vi "Defaults.vi"() -> (3 "TVC Data":T6={"UI References"={"Exit Ref"=refnum, "Save Ref"=refnum, "Export Ref"=refnum, "Acquire Ref"=refnum, "Configure Ref"=refnum, "Graph Ref"=refnum, "Analyze Ref"=refnum, "Status Ref"=refnum, "Snapshot Ref"=refnum, "Start Ref"=refnum}, "User Specified"={"Hardware Configuration"={"VGC50"={"serial settings"={"port"="Inficon_VGC503", "baud rate"=115200}, "device information"={"type"="", "model number"="", "serial number"="", "firmware version"="", "hardware version"=""}, "VGC"=refnum, "Backing SP"={"mode"=2, "thresholds"={"lower"=0.0001, "upper"=0.005}, "on"=FALSE}, "Chamber SP"={"mode"=3, "thresholds"={"lower"=1e-05, "upper"=0.0001}, "on"=FALSE}}, "PTC10"={"serial settings"={"port"="Stanford_PTC10", "baud rate"=9600}, "PTC10 Info"={"Manufacturer"="", "Instrument"="", "Serial Number"="", "Firmware"=""}, "VISA resource name"="", "pwmloop"="define pwmloop(#t=0 while (1) {waitforsample if(#pwm=0){relays=0}else{if(#t<#pwm) {relays=1}else{relays=3}}#t+=1 if  (#t>99){#t=0} pause 0.2 s})", "onecycle"="define onecycle (pwm=100 run pwmloop 5A.PID.Setpoint=-130.0 5A.PID.input=3C while(#3C>-129.0){pause 0.2 s}pwm=-130 pause 10 min pwm=0  5A.PID.SetPoint=50.0 while(#3C<49.0){pause 0.2 s} pause 10 min kill pwmloop)", "control"="define control (while (#Cycles>0) {onecycle pause 1 s #Cycles-=1})", "HeatDrive"="define Failsafe (while(1) {if (#Check <-20){relays=0 outputEnable Off}else{if(#Check>20){relays=0 outputEnable Off}} pause 1 s})", "ToAmbient"="define ToAmbient(if(#3C>25.0){pwm=100 run pwmloop while(#3C>#25.0){pause 0.5 s} pwm=0 kill pwmloop}else{#5A.PID.setpoint=20.0 while(#3C<15.0){pause 0.5 s} outputenable off})", "StartupCode"="system.display.Monitors Show", "LogChannels"=[], "Heater O/P Channel"="", " Control Input"="", "TAmbient"=1.14, "AmbientTolerance"=0.012, "TestCycleParameters"={"TAmb"=20.0, "HeaterTestTemp"=51.5, "HeaterTestDwell(min)"=20, "HeaterTestDuration"=20, "MinOpTemp"=1.0, "MinOpDwell(min)"=1, "TestHeatingRate (deg/min)"=-131.5, "SurviveCycleParameters"={"MinSurviveTemp"=-131.5, "MinSurvive Dwell(min)"=10, "MaxSurviveTemp"=50.0, "MaxSurviveDwell(min)"=30, "ControlInput"=2, "ColdStandOff"=4.0, "HotStandoff"=5.0, "SteadyPWM"=20, "MaxCoolingRate (deg/min)"=3.75, "MaxHeatingRate (deg/min)"=2.5}, "CycleType"=0, "MaxOpTemp"=-50.0, "MinOpDwell(min)"=30}, "PID Params"={"P"=1.14, "I"=0.012, "D"=21.68, "Set"=0.0}}}, "Vacuum Graph config"={"Log/Lin"=FALSE, "Show Backing"=FALSE, "Show Chamber"=FALSE}}} {"User Specified"."Hardware Configuration"."PTC10"."PID Params"."D" min=0.0; "User Specified"."Hardware Configuration"."PTC10"."PID Params"."I" min=0.0; "User Specified"."Hardware Configuration"."PTC10"."PID Params"."P" min=0.0; "User Specified"."Hardware Configuration"."PTC10"."TestCycleParameters"."CycleType" items=["Survival", "Operational"]; "User Specified"."Hardware Configuration"."PTC10"."TestCycleParameters"."SurviveCycleParameters"."SteadyPWM" min=0 max=100 step=1; "User Specified"."Hardware Configuration"."PTC10"."serial settings"."baud rate" items=["9600"=9600, "19200"=19200, "38400"=38400, "57600"=57600, "115200"=115200]; "User Specified"."Hardware Configuration"."VGC50"."Chamber SP"."thresholds"."upper" format="%#_5p"; "User Specified"."Hardware Configuration"."VGC50"."Chamber SP"."thresholds"."lower" format="%#_5p"; "User Specified"."Hardware Configuration"."VGC50"."Chamber SP"."mode" items=["off", "on", "channel 1", "channel 2", "channel 3"]; "User Specified"."Hardware Configuration"."VGC50"."Backing SP"."thresholds"."upper" format="%#_5p"; "User Specified"."Hardware Configuration"."VGC50"."Backing SP"."thresholds"."lower" format="%#_5p"; "User Specified"."Hardware Configuration"."VGC50"."Backing SP"."mode" items=["off", "on", "channel 1", "channel 2", "channel 3"]; "User Specified"."Hardware Configuration"."VGC50"."serial settings"."baud rate" items=["9600"=9600, "19200"=19200, "38400"=38400, "57600"=57600, "115200"=115200]})   [LabVIEW 2024]
uses:
  controls/VGC50.ctl
  <instrlib>/PL Inficon VGC/PL Inficon VGC.lvclass
  controls/Data.ctl
  controls/UI References.ctl
  controls/User Specified Data.ctl
  controls/HW Configuration.ctl
  controls/SRS PTC10.ctl
  controls/TestCycleParams.ctl
  controls/SurviveCycleParams.ctl
  controls/ControlInput.ctl
  controls/PID Params.ctl
  controls/Vac Graph Config.ctl
panel:
  in  "PTC10":T1={"serial settings"={"port"="Stanford_PTC10", "baud rate"=9600}, "PTC10 Info"={"Manufacturer"="", "Instrument"="", "Serial Number"="", "Firmware"=""}, "VISA resource name"="", "pwmloop"="define pwmloop(#t=0 while (1) {waitforsample if(#pwm=0){relays=0}else{if(#t<#pwm) {relays=1}else{relays=3}}#t+=1 if  (#t>99){#t=0} pause 0.2 s})", "onecycle"="define onecycle (pwm=100 run pwmloop 5A.PID.Setpoint=-130.0 5A.PID.input=3C while(#3C>-129.0){pause 0.2 s}pwm=-130 pause 10 min pwm=0  5A.PID.SetPoint=50.0 while(#3C<49.0){pause 0.2 s} pause 10 min kill pwmloop)", "control"="define control (while (#Cycles>0) {onecycle pause 1 s #Cycles-=1})", "HeatDrive"="define Failsafe (while(1) {if (#Check <-20){relays=0 outputEnable Off}else{if(#Check>20){relays=0 outputEnable Off}} pause 1 s})", "ToAmbient"="define ToAmbient(if(#3C>25.0){pwm=100 run pwmloop while(#3C>#25.0){pause 0.5 s} pwm=0 kill pwmloop}else{#5A.PID.setpoint=20.0 while(#3C<15.0){pause 0.5 s} outputenable off})", "StartupCode"="system.display.Monitors Show", "LogChannels"=[], "Heater O/P Channel"="", " Control Input"="", "TAmbient"=20.0, "AmbientTolerance"=5.0, "TestCycleParameters"={"TAmb"=20.0, "HeaterTestTemp"=-80.0, "HeaterTestDwell(min)"=30, "HeaterTestDuration"=15, "MinOpTemp"=-50.0, "MinOpDwell(min)"=30, "TestHeatingRate (deg/min)"=0.4, "SurviveCycleParameters"={"MinSurviveTemp"=-131.5, "MinSurvive Dwell(min)"=10, "MaxSurviveTemp"=50.0, "MaxSurviveDwell(min)"=30, "ControlInput"=2, "ColdStandOff"=4.0, "HotStandoff"=5.0, "SteadyPWM"=20, "MaxCoolingRate (deg/min)"=3.75, "MaxHeatingRate (deg/min)"=2.5}, "CycleType"=0, "MaxOpTemp"=-50.0, "MinOpDwell(min)"=30}, "PID Params"={"P"=1.14, "I"=0.012, "D"=21.68, "Set"=0.0}} {"PID Params"."D" min=0.0; "PID Params"."I" min=0.0; "PID Params"."P" min=0.0; "TestCycleParameters"."CycleType" items=["Survival", "Operational"]; "TestCycleParameters"."SurviveCycleParameters"."SteadyPWM" min=0 max=100 step=1; "TestCycleParameters"."SurviveCycleParameters"."ControlInput" items=["3A", "3B", "3C", "3D", "4A", "4B", "4C", "4D"]; "serial settings"."baud rate" items=["9600"=9600, "19200"=19200, "38400"=38400, "57600"=57600, "115200"=115200]}
  in  "VGC50":T10={"serial settings"={"port"="Inficon_VGC503", "baud rate"=115200}, "device information"={"type"="", "model number"="", "serial number"="", "firmware version"="", "hardware version"=""}, "VGC"=refnum, "Backing SP"={"mode"=2, "thresholds"={"lower"=0.0001, "upper"=0.005}, "on"=FALSE}, "Chamber SP"={"mode"=3, "thresholds"={"lower"=1e-05, "upper"=0.0001}, "on"=FALSE}} {"Chamber SP"."thresholds"."upper" format="%#_5p"; "Chamber SP"."thresholds"."lower" format="%#_5p"; "Chamber SP"."mode" items=["off", "on", "channel 1", "channel 2", "channel 3"]; "Backing SP"."thresholds"."upper" format="%#_5p"; "Backing SP"."thresholds"."lower" format="%#_5p"; "Backing SP"."mode" items=["off", "on", "channel 1", "channel 2", "channel 3"]; "serial settings"."baud rate" items=["9600"=9600, "19200"=19200, "38400"=38400, "57600"=57600, "115200"=115200]}
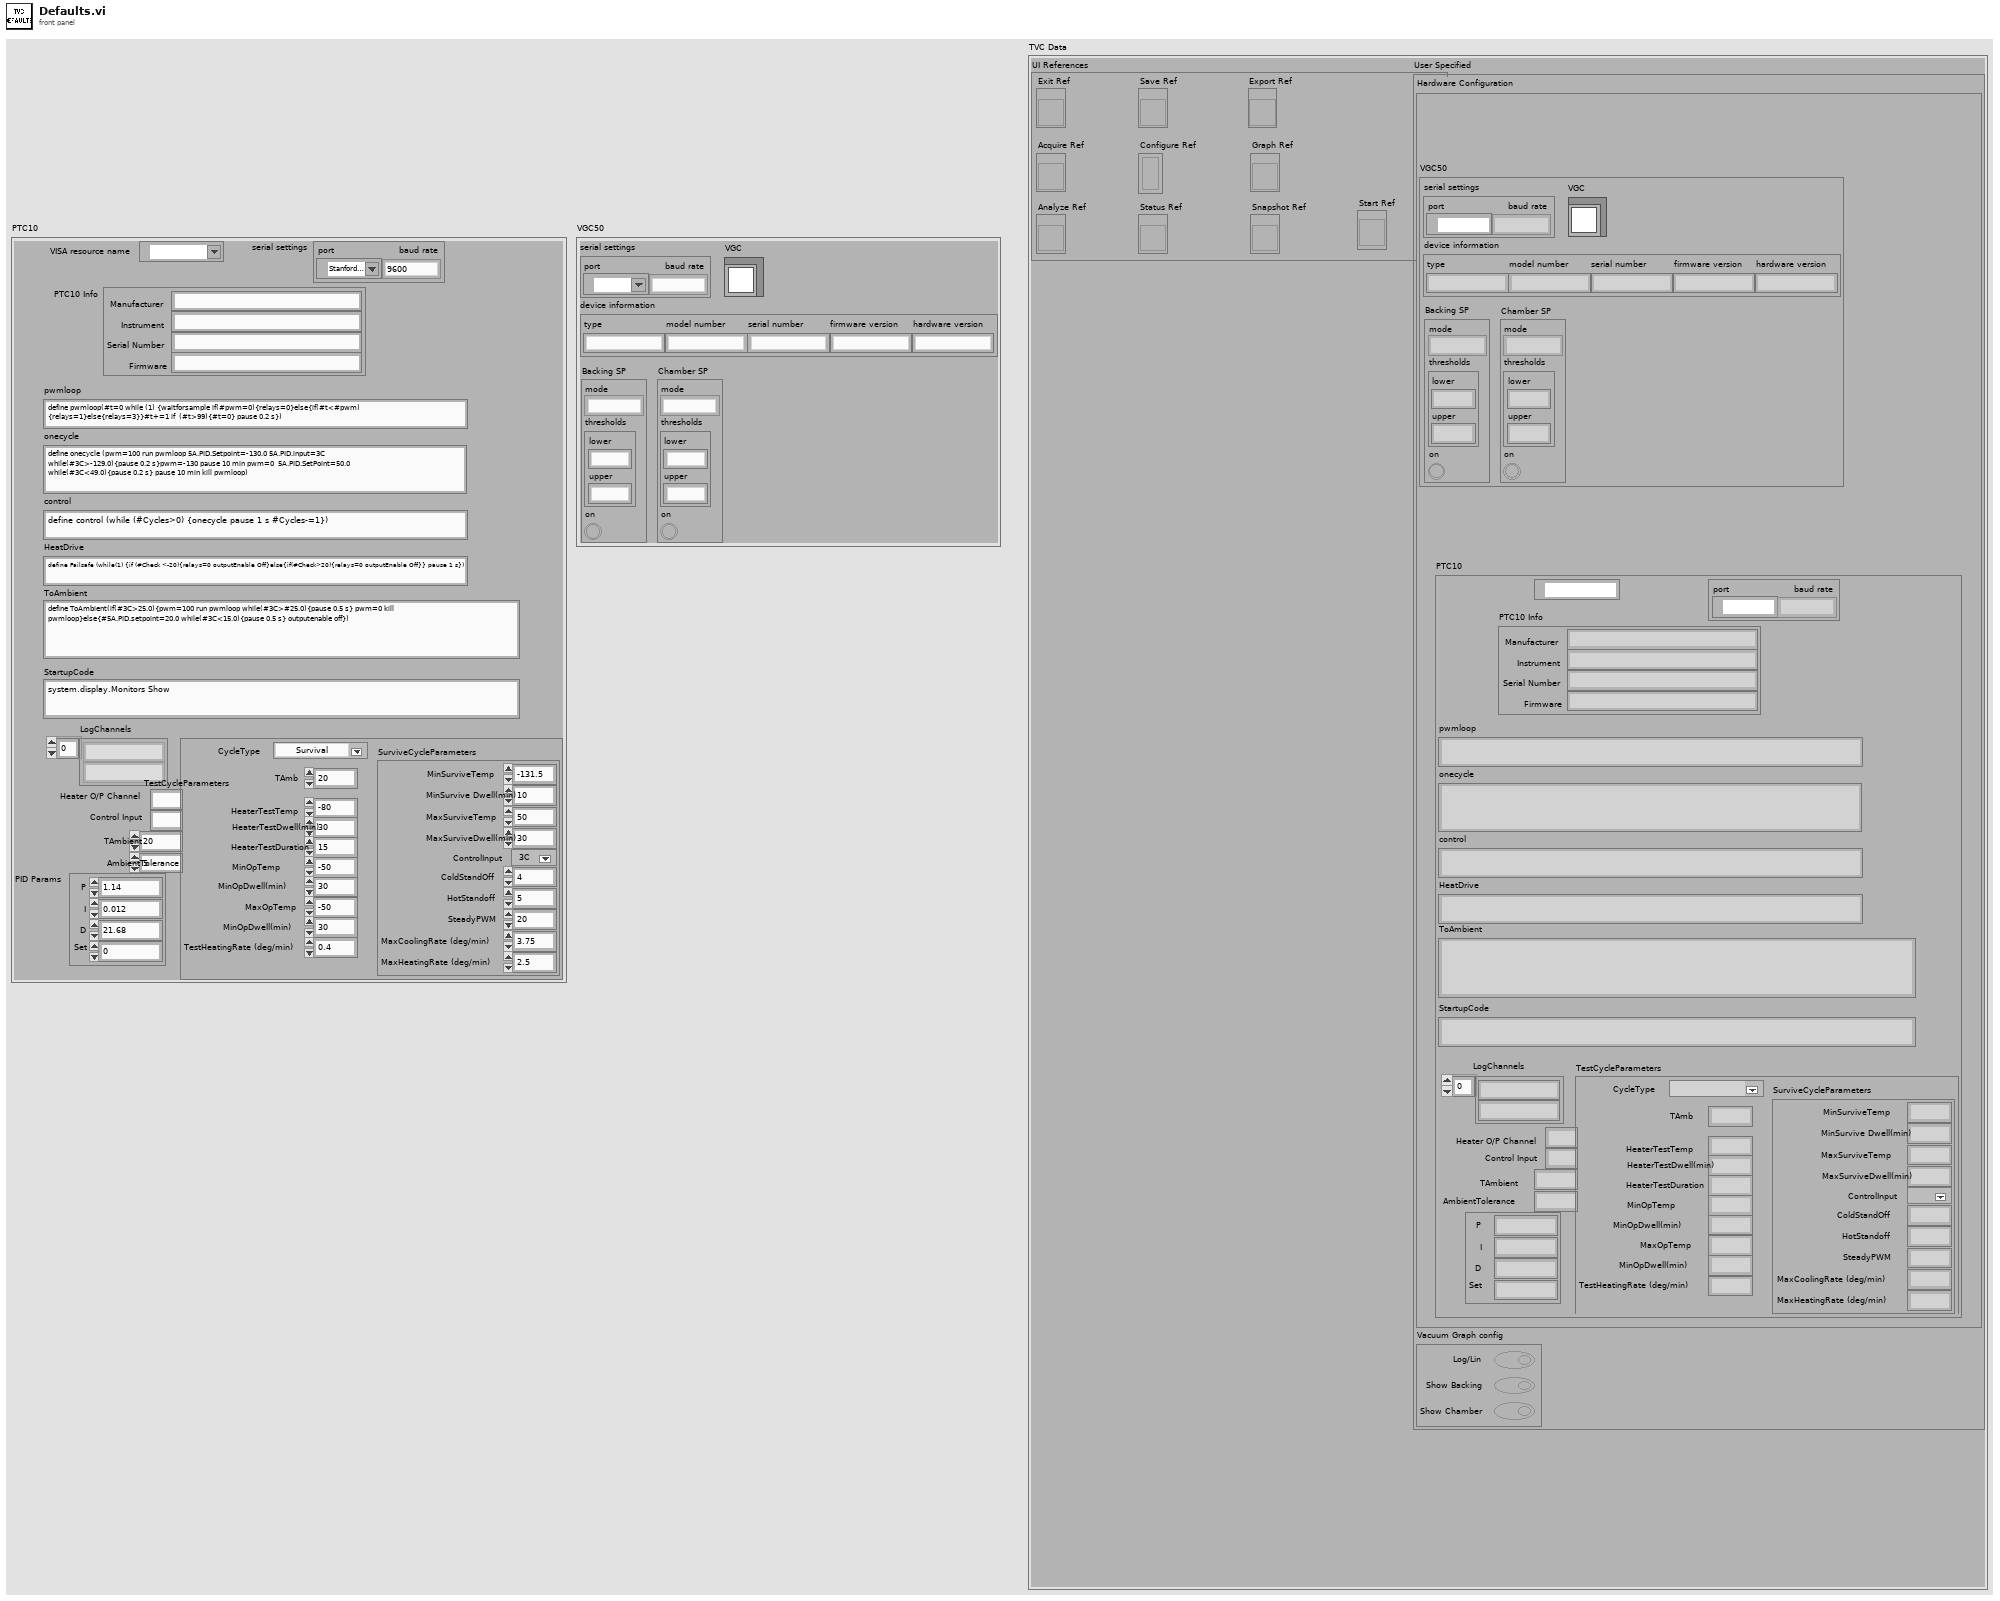
[diagram p1: front panel]
types:
  T1 = typedef "SRS PTC10.ctl" = cluster{"serial settings":cluster{"port":refnum<visa-resource-name>, "baud rate":u32}, "PTC10 Info":cluster{"Manufacturer":string, "Instrument":string, "Serial Number":string, "Firmware":string}, "VISA resource name":refnum<visa-resource-name>, "pwmloop":string, "onecycle":string, "control":string, "HeatDrive":string, "ToAmbient":string, "StartupCode":string, "LogChannels":string[], "Heater O/P Channel":string, " Control Input":string, "TAmbient":dbl, "AmbientTolerance":dbl, "TestCycleParameters":T2, "PID Params":T5}
  T2 = typedef "TestCycleParams.ctl" = cluster{"TAmb":dbl, "HeaterTestTemp":dbl, "HeaterTestDwell(min)":i32, "HeaterTestDuration":i32, "MinOpTemp":dbl, "MinOpDwell(min)":i32, "TestHeatingRate (deg/min)":dbl, "SurviveCycleParameters":T3, "CycleType":u16, "MaxOpTemp":dbl, "MinOpDwell(min)":i32}
  T3 = typedef "SurviveCycleParams.ctl" = cluster{"MinSurviveTemp":dbl, "MinSurvive Dwell(min)":i32, "MaxSurviveTemp":dbl, "MaxSurviveDwell(min)":i32, "ControlInput":T4, "ColdStandOff":dbl, "HotStandoff":dbl, "SteadyPWM":i32, "MaxCoolingRate (deg/min)":dbl, "MaxHeatingRate (deg/min)":dbl}
  T4 = typedef "ControlInput.ctl" = u16
  T5 = typedef "PID Params.ctl" = cluster{"P":dbl, "I":dbl, "D":dbl, "Set":dbl}
  T6 = typedef "Data.ctl" = cluster{"UI References":T7, "User Specified":T8}
  T7 = typedef "UI References.ctl" = cluster{"Exit Ref":refnum<vi>, "Save Ref":refnum<vi>, "Export Ref":refnum<vi>, "Acquire Ref":refnum<vi>, "Configure Ref":refnum<vi>, "Graph Ref":refnum<vi>, "Analyze Ref":refnum<vi>, "Status Ref":refnum<vi>, "Snapshot Ref":refnum<vi>, "Start Ref":refnum<vi>}
  T8 = typedef "User Specified Data.ctl" = cluster{"Hardware Configuration":T9, "Vacuum Graph config":T11}
  T9 = typedef "HW Configuration.ctl" = cluster{"VGC50":T10, "PTC10":T1}
  T10 = typedef "VGC50.ctl" = cluster{"serial settings":cluster{"port":refnum<visa-resource-name>, "baud rate":u32}, "device information":cluster{"type":string, "model number":string, "serial number":string, "firmware version":string, "hardware version":string}, "VGC":refnum<class "PL Inficon VGC.lvclass">, "Backing SP":cluster{"mode":u16, "thresholds":cluster{"lower":dbl, "upper":dbl}, "on":bool}, "Chamber SP":cluster{"mode":u16, "thresholds":cluster{"lower":dbl, "upper":dbl}, "on":bool}}
  T11 = typedef "Vac Graph Config.ctl" = cluster{"Log/Lin":bool, "Show Backing":bool, "Show Chamber":bool}
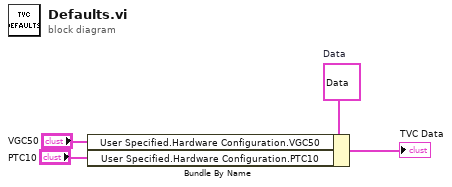
[diagram p0: block diagram]
diagram:
  w4 = T6 {"UI References"={"Exit Ref"=refnum, "Save Ref"=refnum, "Export Ref"=refnum, "Acquire Ref"=refnum, "Configure Ref"=refnum, "Graph Ref"=refnum, "Analyze Ref"=refnum, "Status Ref"=refnum, "Snapshot Ref"=refnum, "Start Ref"=refnum}, "User Specified"={"Hardware Configuration"={"VGC50"={"serial settings"={"port"="Inficon_VGC503", "baud rate"=115200}, "device information"={"type"="", "model number"="", "serial number"="", "firmware version"="", "hardware version"=""}, "VGC"=refnum, "Backing SP"={"mode"=0, "thresholds"={"lower"=0.0, "upper"=0.0}, "on"=FALSE}, "Chamber SP"={"mode"=1, "thresholds"={"lower"=0.0, "upper"=0.0}, "on"=FALSE}}, "PTC10"={"serial settings"={"port"="GPIB0::22::INSTR", "baud rate"=115200}, "PTC10 Info"={"Manufacturer"="", "Instrument"="", "Serial Number"="", "Firmware"=""}, "VISA resource name"="", "pwmloop"="define coldloop(while (1) {if (#3C > -130.0) {relays&=13} if (#3C < -130.0){relays|=2} pause 0.1 s })", "onecycle"="define onecycle (relays=1 while(#3C >-129.0){pause 0.1 s} relays|=2 pause 30 s run\"coldloop\" pause 10 min kill\"coldloop\" relays=4 while(#3C<49.0){pause 0.1 s} pause 10 s run\"hotloop\" pause 10 min kill\"hotloop\" relays=0)", "control"="define control (#count=1 while (#count>0) {onecycle pause 1 s #count-=1})", "HeatDrive"="define coldloop(while (1) {if (#3C > -130.0) {relays&=13} if (#3C < -130.0){relays|=2} pause 0.1 s })", "ToAmbient"="define ToAmbient(if(#3C>25.0){pwm=100 run pwmloop while(#3C>#25.0){pause 0.5 s} pwm=0 kill pwmloop}else{#5A.PID.setpoint=20.0 while(#3C<15.0){pause 0.5 s} outputenable off})", "StartupCode"="system.display.Monitors Show", "LogChannels"=[], "Heater O/P Channel"="", " Control Input"="", "TAmbient"=20.0, "AmbientTolerance"=5.0, "TestCycleParameters"={"TAmb"=20.0, "HeaterTestTemp"=20.0, "HeaterTestDwell(min)"=1, "HeaterTestDuration"=1, "MinOpTemp"=-131.5, "MinOpDwell(min)"=30, "TestHeatingRate (deg/min)"=0.4, "SurviveCycleParameters"={"MinSurviveTemp"=-131.5, "MinSurvive Dwell(min)"=10, "MaxSurviveTemp"=50.0, "MaxSurviveDwell(min)"=30, "ControlInput"=2, "ColdStandOff"=4.0, "HotStandoff"=5.0, "SteadyPWM"=20, "MaxCoolingRate (deg/min)"=3.75, "MaxHeatingRate (deg/min)"=2.5}, "CycleType"=0, "MaxOpTemp"=-50.0, "MinOpDwell(min)"=30}, "PID Params"={"P"=1.14, "I"=0.012, "D"=21.68, "Set"=0.0}}}, "Vacuum Graph config"={"Log/Lin"=FALSE, "Show Backing"=FALSE, "Show Chamber"=FALSE}}}  # Data
  n1 = Bundle By Name(cluster=w4, "User Specified.Hardware Configuration.VGC50"="VGC50", "User Specified.Hardware Configuration.PTC10"="PTC10") -> (→"TVC Data":T6)
